vi "FPGA.vi"   [LabVIEW 2019]
uses:
  <vilib>/rvi/Emulation/niFpgaGetClockAttributes.vi
  <vilib>/rvi/Emulation/niFpgaSctlEmulationGetInTimedLoop.vi
  <vilib>/rvi/Emulation/niFpgaEmulationReportErrorSimple.vi
  <vilib>/rvi/eio/common/nirviEmuTemplateMethod_errors.vi
  <vilib>/rvi/eio/common/nirviEmuTemplatePropertyGet_noerrors.vi
  <vilib>/rvi/eio/common/nirviEmuTemplatePropertySet_noerrors.vi
  <vilib>/rvi/Emulation/niFpgaCriticalErrorInLSC.vi
  <vilib>/eio/EIONode/EIONode.xnode
  <vilib>/eio/EIOMethodNode/EIOMethodNode.xnode
  <vilib>/eio/EIOPropertyNode/EIOPropertyNode.xnode
  <vilib>/LabVIEW Targets/FPGA/cRIO/cRIO-9505/controls.llb/_nicrio_cRIO-9505_DriveStatus.ctl
  <vilib>/LabVIEW Targets/FPGA/cRIO/cRIO-9505/controls.llb/_nicrio_cRIO-9505_DriveDirection.ctl
  <vilib>/rvi/eio/common/nirviEmuTemplatePropertyGet_errors.vi
  <vilib>/rvi/eio/common/nirviEmuTemplatePropertySet_errors.vi
types:
  T1 = typedef "_nicrio_cRIO-9505_DriveStatus.ctl" = enum8{"Enabled", "Disabled", "Disabled by Drive Fault", "Disabled by Temp. Fault", "Disabled by E-Stop", "Unknown"}
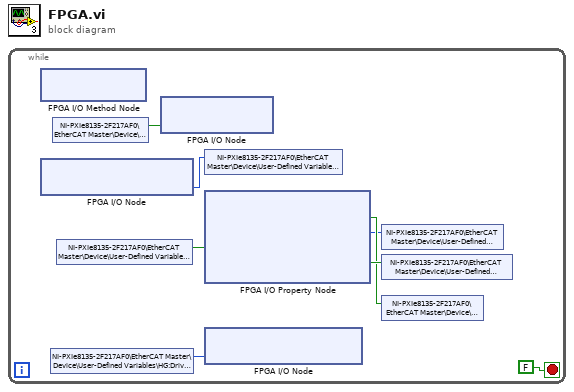
[diagram p0: block diagram]
diagram:
  n1 = while {
    stop <- FALSE stop-if-true
    n2 = xnode "FPGA I/O Method Node"() -> ()  [unwired: 1 in, 1 out]
    n3 = xnode "FPGA I/O Node"() -> ("Mod5/Current Sense"=w1:i16)  [unwired: 1 in, 1 out]
    n4 = shared-variable "NI-PXIe8135-2F217AF0\\EtherCAT Master\\Device\\User-Defined Variables\\HG:Drive Direction"() -> (w2:i16)  [unwired: 1 in, 1 out]
    n5 = shared-variable "NI-PXIe8135-2F217AF0\\EtherCAT Master\\Device\\User-Defined Variables\\HF:Motor"() -> (w8:bool)  [unwired: 1 in, 1 out]
    n6 = shared-variable "NI-PXIe8135-2F217AF0\\EtherCAT Master\\Device\\User-Defined Variables\\HF:Enable E-Stop"() -> (w3:bool)  [unwired: 1 in, 1 out]
    n7 = xnode "FPGA I/O Node"("Mod5/Motor"=w8) -> ()  [unwired: 1 in, 1 out]
    n8 = shared-variable "NI-PXIe8135-2F217AF0\\EtherCAT Master\\Device\\User-Defined Variables\\GH:Current Sense"(w1) -> ()  [unwired: 1 in, 1 out]
    n9 = xnode "FPGA I/O Property Node"("Enable E-Stop"=w3) -> ("Drive Fault"=w5:bool, "Drive Status"=w4:T1, "Vsup Present"=w7:bool)  [unwired: 1 in, 2 out]
    n10 = xnode "FPGA I/O Node"("Mod5/Drive Direction"=w2) -> ()  [unwired: 1 in, 1 out]
    n11 = shared-variable "NI-PXIe8135-2F217AF0\\EtherCAT Master\\Device\\User-Defined Variables\\FH:DriveStatus"(w4) -> ()  [unwired: 1 in, 1 out]
    n12 = shared-variable "NI-PXIe8135-2F217AF0\\EtherCAT Master\\Device\\User-Defined Variables\\FH:Vsup Present"(w7) -> ()  [unwired: 1 in, 1 out]
    n13 = shared-variable "NI-PXIe8135-2F217AF0\\EtherCAT Master\\Device\\User-Defined Variables\\FH:DriveFa"(w5) -> ()  [unwired: 1 in, 1 out]
  }
